vi "cluster_v1.vi"() -> ()   [LabVIEW 2009]
panel:
  in  "stop":bool
  in  "Delta t":dbl(slide) scale=0.0..10.0
  out "Waveform Graph":cluster{"Slide":i32, "Slide 2":dbl, u16[]}(graph)
  in  "to":i32(slide) scale=0.0..10.0
  out "Array":dbl[](array[numeric])
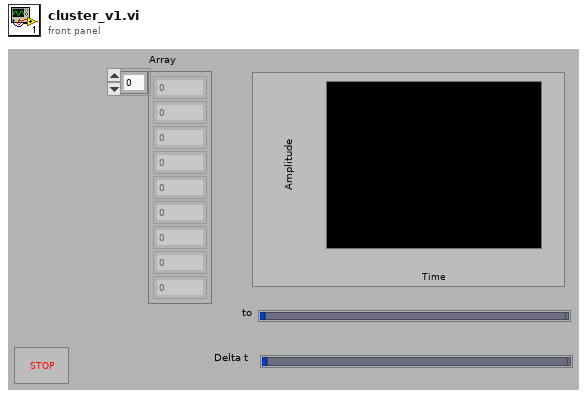
[diagram p1: front panel]
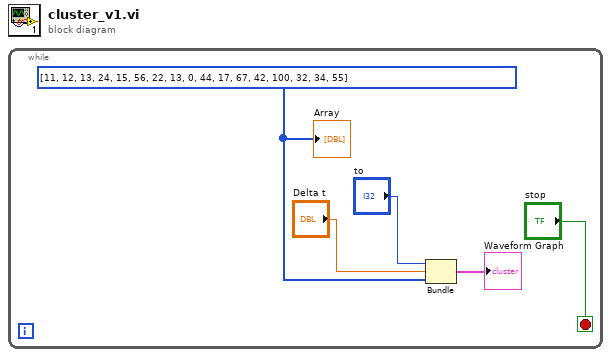
[diagram p0: block diagram]
diagram:
  n1 = while {
    stop <- "stop" stop-if-true
    w5 = u16[] [11, 12, 13, 24, 15, 56, 22, 13, 0, 44, 17, 67, 42, 100, 32, 34, 55]
    n2 = Bundle("to"="to", "Delta t"="Delta t", w5) -> (→"Waveform Graph":cluster{"to":i32, "Delta t":dbl, u16[]})  [unwired: 1 in]
    "Array" <- w5
  }
